vi "MyDLMagnetInitialize (SubVI).vi"(8 "error in":errorcluster, 11 "VISA resource name in":refnum<visa-resource-name>) -> (0 "error out":errorcluster, 3 "VISA Refnum out":refnum<visa-resource-name>)   [LabVIEW 2025, in "MyTriton.lvlib"]
uses:
  MyTriton.lvlib
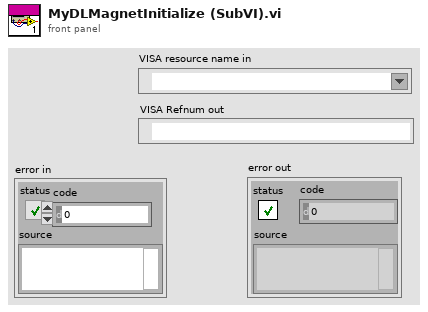
[diagram p1: front panel]
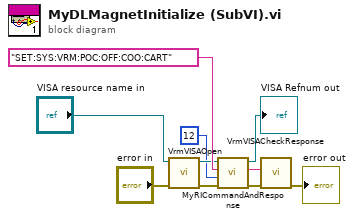
[diagram p0: block diagram]
diagram:
  n1 = call "VrmVISAOpen.vi"("error in (no error)"="error in", "VISA resource name in"="VISA resource name in") -> ("error out"=w7:errorcluster, "VISA resource name out"=w8:refnum<visa-resource-name>)  [unwired: 8 in]
  n2 = call "MyRICommandAndResponse.vi"("error in (no error)"=w7, "Min byte count"=u32 12, "Command"="SET:SYS:VRM:POC:OFF:COO:CART", "VISA resource name in"=w8) -> ("error out"=w4:errorcluster, "Response"=w5:string, "VISA resource name out"=→"VISA Refnum out":refnum<visa-resource-name>)  [unwired: 5 in]
  n3 = call "VrmVISACheckResponse.vi"("error in (no error)"=w4, "Response"=w5) -> ("error out"=→"error out":errorcluster)  [unwired: 8 in, 1 out]
